vi "Load_from_Project.vi"(8 "error in (no error)":errorcluster, 9 "index":i32, 10 "buildObject":T3, 11 "AB_Source_ExportedVI in":refnum<class "AB_Source_ExportedVI.lvclass">) -> (0 "error out":errorcluster, 2 "linker info":T2, 3 "AB_Source_ExportedVI out":refnum<class "AB_Source_ExportedVI.lvclass">)   [LabVIEW 2020, in "AB_Source_ExportedVI.lvclass"]
uses:
  <vilib>/AppBuilder/AB_Classes/Source/ExportedVI/AB_Source_ExportedVI.lvclass
  <resource>/Framework/Providers/API/ItemRef.ctl
  <vilib>/Utility/lvfile.llb/LVFileType.ctl
  <vilib>/AppBuilder/RW_Project/AB_RW_Project_PropBag_Action.ctl
  <vilib>/AppBuilder/AB_Classes/Source/ExportedVI/AB_Source_ExportedVI.lvclass/AB_Source_ExportedVI.ctl
  <vilib>/AppBuilder/AB_Classes/Source/VI/AB_Source_VI.lvclass
  <vilib>/Utility/lvfile.llb/NI_FileType.lvlib
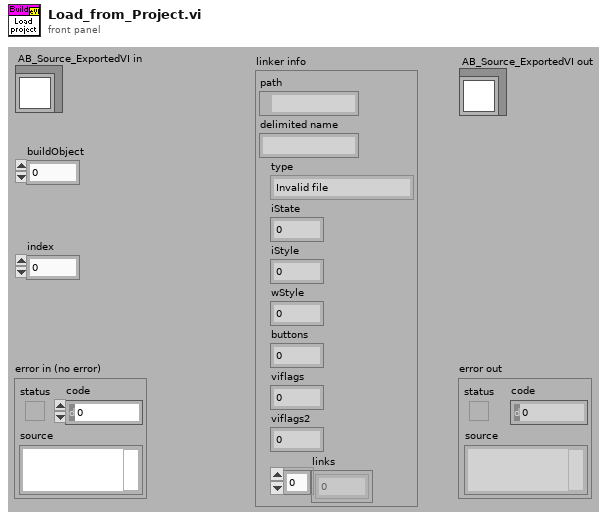
[diagram p1: front panel]
types:
  T1 = typedef "NI_FileType.lvlib/LVFileType.ctl" = enum32{"Invalid file", "Unknown type", "Instrument", "Control", "Polymorphic VI", "Project", "Library", "LVClass", "XControl", "XNode", "Shared library", ".NET assembly", "ActiveX interface", "CIN", "Run-time menu", "Palette menu", "Help file", "LLB", "XNode Edit Dependency", "Class Private Data Control", "Statechart", "MathScript .m file", "Ladder Diagram", "LVLibp", "XNode Build Dependency"}
  T2 = cluster{"path":path, "delimited name":string, "type":T1, "iState":u32, "iStyle":u16, "wStyle":u16, "buttons":u16, "viflags":u32, "viflags2":u32, "links":u32[]}
  T3 = typedef "ItemRef.ctl" = u64
  T4 = typedef "AB_RW_Project_PropBag_Action.ctl" = enum16{"read", "write", "clear", "readPrevious", "writePrevious", "clearPrevious"}
  T5 = typedef "AB_RW_Project_Source_ExportedVI_Data_New.ctl" = cluster{"vipInfo":T6}
  T6 = typedef "ABAPI Dist VI Proto Info New.ctl" = cluster{"cptm":string, "params":cluster{"name":string, "dir":enum32{"in", "out", "in/out", "length", "error-out"}, "inputIdx":i32, "outputIdx":i32, "passBy":i32, "lenInput":i32, "lenOutput":i32}[], "callingConv":i32, "name":string, "Description":string, "isCustomDesc":i32}
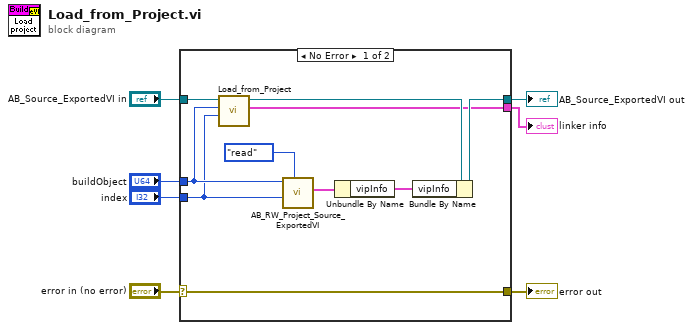
[diagram p0: block diagram]
diagram:
  n1 = case shown="No Error" "error in (no error)" {
    selector: "error in (no error)" -> [w16 w18]
    tunnel: "AB_Source_ExportedVI in" -> [w17 w19]
    tunnel: [w11 w19] -> w5
    tunnel: [w16 w18] -> w4
    tunnel: "buildObject" -> [w15 _]
    tunnel: "index" -> [w14 _]
    tunnel: [w8 _] -> w1
    frame No Error {
      n2 = call-parent "Load_from_Project.vi"("index"=w14, "buildObject"=w15, "AB_Source_VI in"=w17) -> ("linker info"=w8:T2, "AB_Source_VI out"=w12:refnum<class "AB_Source_ExportedVI.lvclass">)  [unwired: 6 in, 1 out]
      n3 = call <vilib>:"AB_RW_Project_Source_ExportedVI.vi"("action"=AB_RW_Project_PropBag_Action."read", "index in"=w14, "buildObject"=w15) -> ("dataSource out"=w10:T5)  [unwired: 5 in, 3 out]
      n4 = Unbundle By Name(w10) -> ("vipInfo"=w9:T6)
      n5 = Bundle By Name(cluster=w12, "vipInfo"=w9) -> (w11:refnum<class "AB_Source_ExportedVI.lvclass">)
    }
    frame Error {
    }
  }
  "error out" <- w4
  "AB_Source_ExportedVI out" <- w5
  "linker info" <- w1
